vi "3D Quadrature Formula Str Func.vi"(8 "data":variant, 9 "Z":dbl[](array[numeric]), 10 "Y":dbl[](array[numeric]), 11 "X":dbl[](array[numeric])) -> (0 "error out":errorcluster, 3 "F(X,Y,Z)":dbl[](array[numeric]))   [LabVIEW 2020, in "NI_AALPro.lvlib"]
uses:
  NI_AALPro.lvlib
  NI_Gmath.lvlib
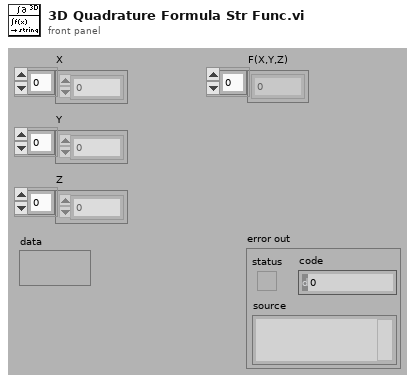
[diagram p1: front panel]
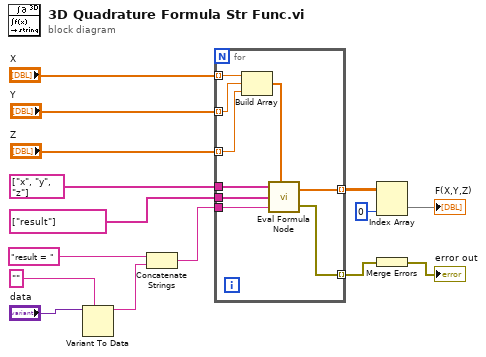
[diagram p0: block diagram]
diagram:
  n1 = Variant To Data(type="" ("string"), Variant="data") -> (data=w8:string)  [unwired: 1 in, 1 out]
  n2 = Concatenate Strings("result = " ("string"), w8) -> (w14:string)
  n3 = for {
    tunnel: w14 -> [w24]
    tunnel: string[] ["result"] ("Variables Output") -> [w23]
    tunnel: string[] ["x", "y", "z"] ("Variables Output") -> [w22]
    tunnel: "X" -> [w21] mode=indexing
    tunnel: [w19] -> w5 mode=indexing
    tunnel: [w18] -> w6 mode=indexing
    tunnel: "Y" -> [w17] mode=indexing
    tunnel: "Z" -> [w16] mode=indexing
    n4 = Build Array(w21, w17, w16) -> (w20:dbl[])
    n5 = call "Eval Formula Node.vi"("Variables Input"=w22, "Input Values"=w20, "Variables Output"=w23, "formula"=w24) -> ("Output Values"=w19:dbl[], "error out"=w18:errorcluster)  [unwired: 1 in]
  }
  n6 = Index Array(array=w5, index (col)=0 ("disabled index (col)")) -> (element=→"F(X,Y,Z)":dbl[])  [unwired: 1 in]
  n7 = Merge Errors(w6) -> (→"error out":errorcluster)
